vi "S7.vi"() -> ()   [LabVIEW 2018]
panel:
  out "value":bool
  in  "address":string
  in  "write":bool[](array[boolean])
  out "Close?":bool
  in  "停止":bool
  out "IsSuccess":bool
  in  "ipAddress":string
  in  "siemens":i32(ring)=1 items=["S1200"=1, "S300"=2, "S400"=3, "S1500"=4, "S200Smart"=5, "S200"=6]
  # "S7"
  # "read"
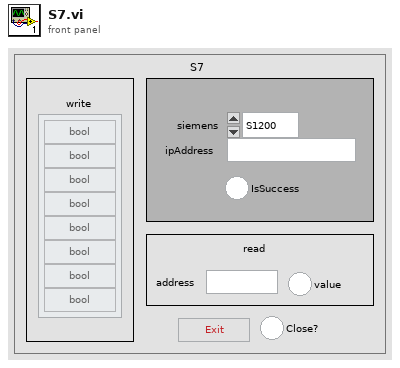
[diagram p1: front panel]
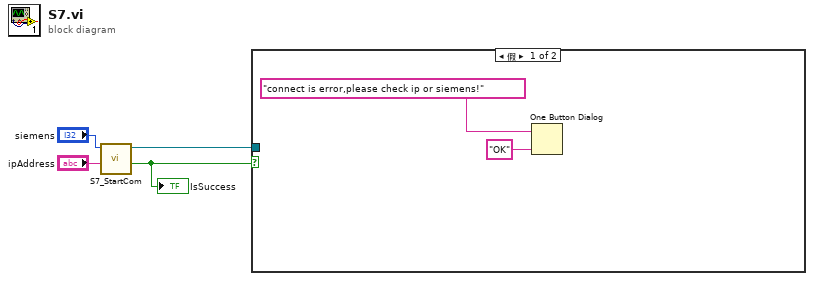
[diagram p0: block diagram]
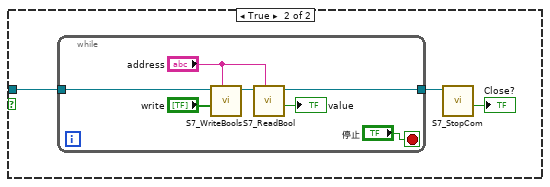
[diagram p2: hidden frame]
diagram:
  n1 = call "S7_StartCom.vi"("ipAddress"="ipAddress", "siemens"="siemens") -> ("IsSuccess"=w1:bool, "connect id"=w4:refnum<k24>)  [unwired: 7 in, 1 out]
  "IsSuccess" <- w1
  n2 = case shown="假" w1 {
    tunnel: w4 -> [_ w9]
    frame False {
      n3 = One Button Dialog(message="connect is error,please check ip or siemens!" ("消息"), button name ("OK")="OK" ("按钮名称（“确定”）")) -> ()  [unwired: 1 out]
    }
    frame True {
      n4 = while {
        tunnel: w9 -> [w15]
        tunnel: [w11] -> w8
        stop <- "停止" stop-if-true
        n5 = call "S7_WriteBools.vi"("address"="address", "values"="write", "connect id"=w15) -> ("connect id"=w13:refnum<k24>)  [unwired: 5 in, 3 out]
        n6 = call "S7_ReadBool.vi"("address"="address", "connect id"=w13) -> ("value"=→"value":bool, "connect id"=w11:refnum<k24>)  [unwired: 6 in, 2 out]
      }
      n7 = call "S7_StopCom.vi"("connect id"=w8) -> ("IsSuccess"=→"Close?":bool)  [unwired: 8 in, 2 out]
    }
  }
